vi "Threshold Checker.vi"(9 "start index (0)":i32, 10 "Threshold":dbl, 11 "Data":dbl[](array[numeric])) -> (1 "buffer filled?":bool, 2 "Index of Value = to or exceeding threshold":i32, 3 "Did we pass the threshold?":bool)   [LabVIEW 2014]
panel:
  in  "Number of buffer points":dbl
  # "Threshold Checker VI"
  # "Inputs"
  # "Outputs"
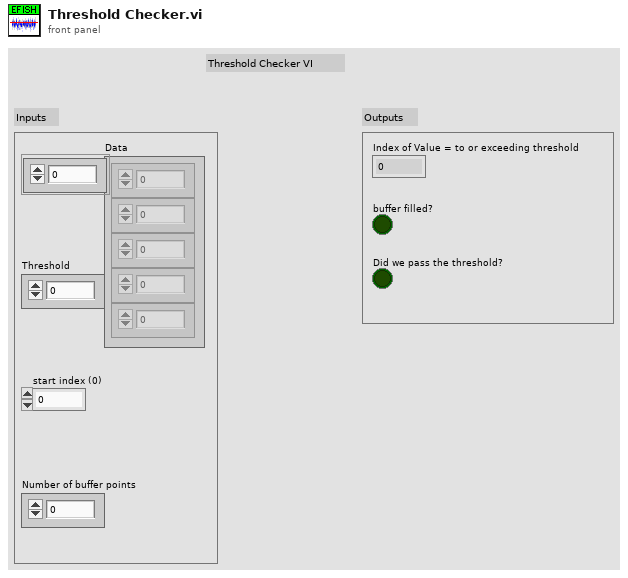
[diagram p1: front panel]
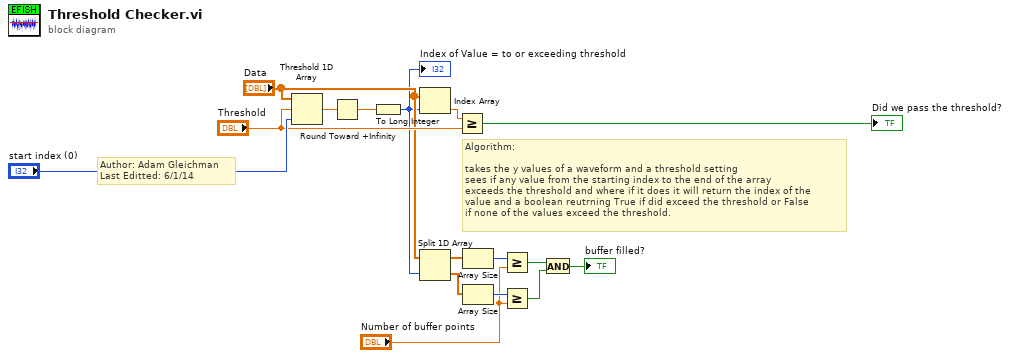
[diagram p0: block diagram]
diagram:
  # "Author: Adam Gleichman\nLast Editted: 6/1/14"
  # "Algorithm:\n\ntakes the y values of a waveform and a threshold setting\nsees if any value from the starting index to the end of the array \nexceeds the threshold and where if it does it will return the index of the\nvalue and a boolean reutrning True if did exceed the threshold or False\nif none of the values exceed the threshold."
  n1 = Threshold 1D Array(1:"start index (0)", 2:"Threshold", 3:"Data") -> (0:w3:dbl)
  n2 = Round Toward +Infinity(x=w3) -> (ceil(x): smallest int >= x=w2:dbl)
  n3 = To Long Integer(number=w2) -> (32bit integer=w1:i32)
  "Index of Value = to or exceeding threshold" <- w1
  n4 = Index Array(array="Data", index=w1) -> (element=w15:dbl)
  n5 = Split 1D Array(array="Data", index=w1) -> (first subarray=w9:dbl[], second subarray=w10:dbl[])
  n6 = Greater Or Equal?(x=w15, y="Threshold") -> (x >= y?=→"Did we pass the threshold?":bool)
  n7 = Array Size(array=w9) -> (size(s)=w8:i32)
  n8 = Array Size(array=w10) -> (size(s)=w11:i32)
  n9 = Greater Or Equal?(x=w8, y="Number of buffer points") -> (x >= y?=w5:bool)
  n10 = Greater Or Equal?(x=w11, y="Number of buffer points") -> (x >= y?=w6:bool)
  n11 = And(x=w5, y=w6) -> (x .and. y?=→"buffer filled?":bool)
